vi "serialization tests.vi"() -> (0 "validation error":errorcluster, 1 "modules equal":bool, 4 "serialization error":errorcluster, 5 "channels equal":bool)   [LabVIEW 2015, in "SystemLink File Module tests.lvlib"]
doc: "Tests the 'To String' and 'From String' methods of the Module's configuration class and ensures they are compatible."
uses:
  SystemLink File Module tests.lvlib
  module/configuration/SystemLink File configuration.lvclass
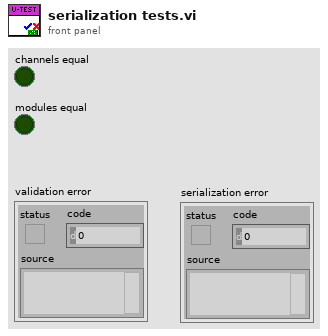
[diagram p1: front panel]
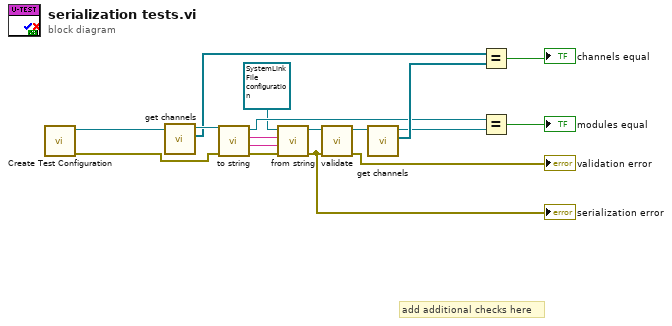
[diagram p0: block diagram]
diagram:
  # "add additional checks here"
  n1 = call "Create Test Configuration.vi"() -> ("error out"=w1:errorcluster, "Module Configuration"=w2:refnum<class "SystemLink File configuration.lvclass">)  [unwired: 7 in, 3 out]
  n2 = call-dynamic "get channels.vi"("SystemLin Tag Module configuration in"=w2) -> ("channels"=w4:refnum<class "TBM channel.lvclass">[], "SystemLin Tag Module configuration out"=w5:refnum<class "SystemLink File configuration.lvclass">)  [unwired: 9 in]
  n3 = call-dynamic "to string.vi"("error in"=w1, "SystemLin Tag Module configuration in"=w5) -> ("error out"=w17:errorcluster, "data"=w16:string, "version"=w15:string, "SystemLin Tag Module configuration out"=w7:refnum<class "SystemLink File configuration.lvclass">)  [unwired: 6 in]
  n4 = call-dynamic "from string.vi"("error in"=w17, "data"=w16, "version"=w15, "SystemLin Tag Module configuration in"=refnum<class "SystemLink File configuration.lvclass"> refnum ("tag bus configurable plugin module configuration")) -> ("error out"=w12:errorcluster, "SystemLin Tag Module configuration out"=w14:refnum<class "SystemLink File configuration.lvclass">)  [unwired: 6 in]
  "serialization error" <- w12
  n5 = call-dynamic "validate.vi"("error in"=w12, "SystemLin Tag Module configuration in"=w14) -> ("error out"=→"validation error":errorcluster, "SystemLin Tag Module configuration out"=w10:refnum<class "SystemLink File configuration.lvclass">)  [unwired: 8 in]
  n6 = call-dynamic "get channels.vi"("SystemLin Tag Module configuration in"=w10) -> ("channels"=w9:refnum<class "TBM channel.lvclass">[], "SystemLin Tag Module configuration out"=w3:refnum<class "SystemLink File configuration.lvclass">)  [unwired: 9 in]
  n7 = Equal?(x=w4, y=w9) -> (x = y?=→"channels equal":bool)
  n8 = Equal?(x=w7, y=w3) -> (x = y?=→"modules equal":bool)
